vi "watt_decluster_by_time.vi"(9 "t_final":dbl format="%_19f", 10 "t_init":dbl format="%_19f", 11 "watt array cluster":T1) -> (2 "Dados":dbl[][](array[numeric]), 3 "Tempo":dbl[](array[numeric]))   [LabVIEW 2019]
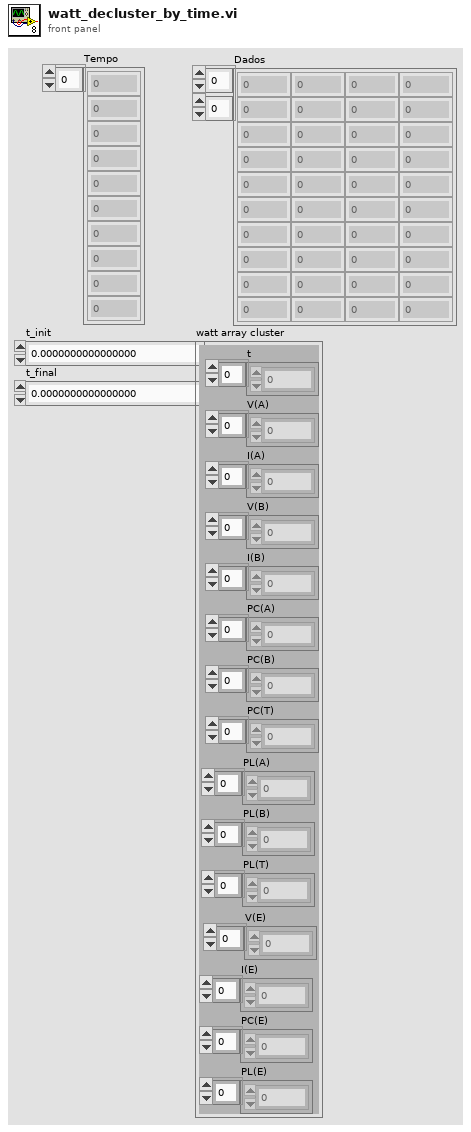
[diagram p1: front panel]
types:
  T1 = cluster{"t":dbl[], "V(A)":dbl[], "I(A)":dbl[], "V(B)":dbl[], "I(B)":dbl[], "PC(A)":dbl[], "PC(B)":dbl[], "PC(T)":dbl[], "PL(T)":dbl[], "PL(B)":dbl[], "PL(A)":dbl[], "V(E)":dbl[], "PL(E)":dbl[], "PC(E)":dbl[], "I(E)":dbl[]}
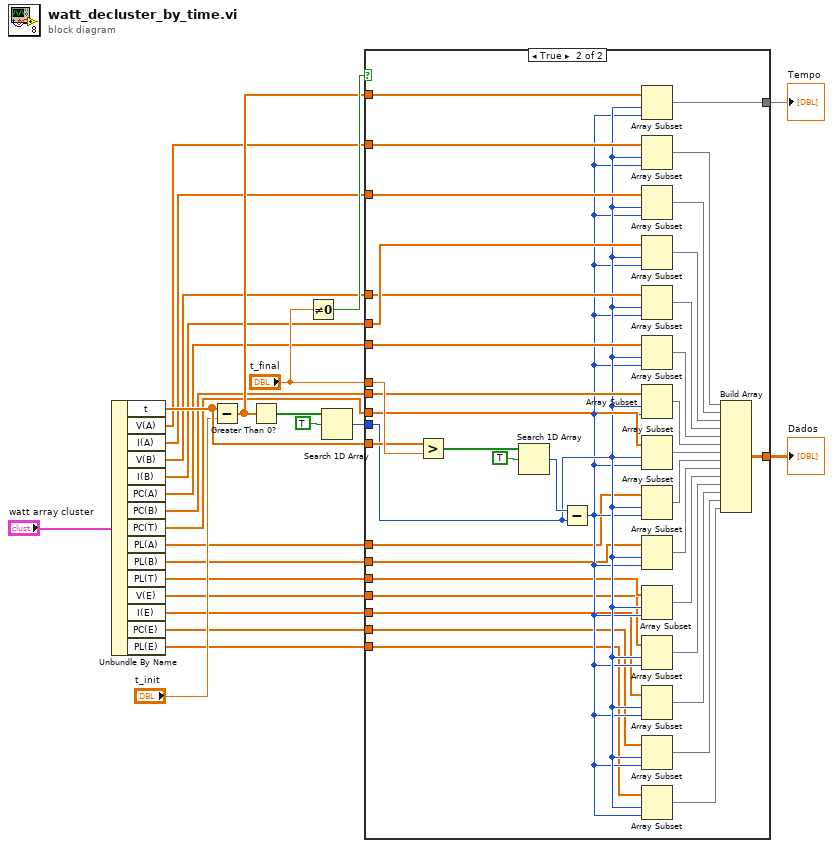
[diagram p0: block diagram]
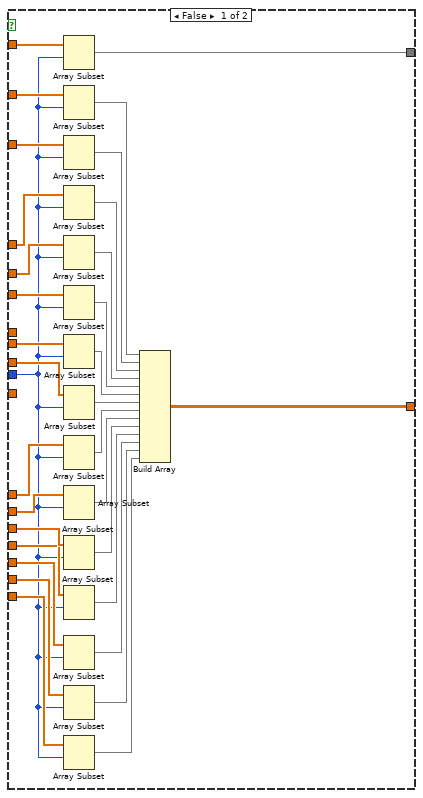
[diagram p2: hidden frame]
diagram:
  n1 = Unbundle By Name("watt array cluster") -> ("t"=w19:dbl[], "V(A)"=w13:dbl[], "I(A)"=w14:dbl[], "V(B)"=w16:dbl[], "I(B)"=w15:dbl[], "PC(A)"=w11:dbl[], "PC(B)"=w10:dbl[], "PC(T)"=w9:dbl[], "PL(A)"=w7:dbl[], "PL(B)"=w6:dbl[], "PL(T)"=w5:dbl[], "V(E)"=w4:dbl[], "I(E)"=w3:dbl[], "PC(E)"=w2:dbl[], "PL(E)"=w1:dbl[])
  n2 = Subtract(x=w19, y="t_init") -> (x-y=w22:dbl[])
  n3 = Greater Than 0?(x=w22) -> (x > 0?=w24:bool[])
  n4 = Not Equal To 0?(x="t_final") -> (x != 0?=w23:bool)
  n5 = Search 1D Array(1D array=w24, element=TRUE) -> (index of element=w21:i32)  [unwired: 1 in]
  n6 = case shown="True" w23 {
    tunnel: w22 -> [w57 w95]
    tunnel: w21 -> [w33 w73]
    tunnel: [w56 w94] -> w20
    tunnel: "t_final" -> [_ w90]
    tunnel: w19 -> [_ w89]
    tunnel: w16 -> [w51 w81]
    tunnel: w15 -> [w50 w82]
    tunnel: w14 -> [w49 w83]
    tunnel: w13 -> [w48 w84]
    tunnel: [w47 w80] -> w12
    tunnel: w11 -> [w46 w79]
    tunnel: w10 -> [w45 w78]
    tunnel: w9 -> [w44 w77]
    tunnel: w7 -> [w40 w71]
    tunnel: w6 -> [w39 w70]
    tunnel: w5 -> [w38 w69]
    tunnel: w4 -> [w37 w68]
    tunnel: w3 -> [w36 w67]
    tunnel: w2 -> [w35 w66]
    tunnel: w1 -> [w34 w65]
    frame False {
      n7 = Array Subset(array=w57, index=w33) -> (w56:dbl[])  [unwired: 1 in]
      n8 = Array Subset(array=w48, index=w33) -> (w52:dbl[])  [unwired: 1 in]
      n9 = Array Subset(array=w49, index=w33) -> (w53:dbl[])  [unwired: 1 in]
      n10 = Array Subset(array=w51, index=w33) -> (w54:dbl[])  [unwired: 1 in]
      n11 = Array Subset(array=w50, index=w33) -> (w55:dbl[])  [unwired: 1 in]
      n12 = Array Subset(array=w46, index=w33) -> (w43:dbl[])  [unwired: 1 in]
      n13 = Array Subset(array=w45, index=w33) -> (w42:dbl[])  [unwired: 1 in]
      n14 = Array Subset(array=w44, index=w33) -> (w41:dbl[])  [unwired: 1 in]
      n15 = Array Subset(array=w40, index=w33) -> (w32:dbl[])  [unwired: 1 in]
      n16 = Array Subset(array=w39, index=w33) -> (w31:dbl[])  [unwired: 1 in]
      n17 = Array Subset(array=w38, index=w33) -> (w30:dbl[])  [unwired: 1 in]
      n18 = Array Subset(array=w37, index=w33) -> (w29:dbl[])  [unwired: 1 in]
      n19 = Array Subset(array=w36, index=w33) -> (w28:dbl[])  [unwired: 1 in]
      n20 = Array Subset(array=w35, index=w33) -> (w27:dbl[])  [unwired: 1 in]
      n21 = Array Subset(array=w34, index=w33) -> (w26:dbl[])  [unwired: 1 in]
      n22 = Build Array(w52, w53, w54, w55, w43, w42, w41, w32, w31, w30, w29, w28, w27, w26) -> (w47:dbl[][])
    }
    frame True {
      n23 = Greater?(x=w89, y=w90) -> (0:w92:bool[])
      n24 = Search 1D Array(1D array=w92, element=TRUE) -> (index of element=w93:i32)  [unwired: 1 in]
      n25 = Subtract(x=w93, y=w73) -> (x-y=w72:i32)
      n26 = Array Subset(array=w95, index=w73, length=w72) -> (w94:dbl[])
      n27 = Array Subset(array=w84, index=w73, length=w72) -> (w85:dbl[])
      n28 = Array Subset(array=w83, index=w73, length=w72) -> (w86:dbl[])
      n29 = Array Subset(array=w82, index=w73, length=w72) -> (w87:dbl[])
      n30 = Array Subset(array=w81, index=w73, length=w72) -> (w88:dbl[])
      n31 = Array Subset(array=w79, index=w73, length=w72) -> (w76:dbl[])
      n32 = Array Subset(array=w78, index=w73, length=w72) -> (w75:dbl[])
      n33 = Array Subset(array=w77, index=w73, length=w72) -> (w74:dbl[])
      n34 = Array Subset(array=w71, index=w73, length=w72) -> (w64:dbl[])
      n35 = Array Subset(array=w70, index=w73, length=w72) -> (w63:dbl[])
      n36 = Array Subset(array=w69, index=w73, length=w72) -> (w62:dbl[])
      n37 = Array Subset(array=w68, index=w73, length=w72) -> (w61:dbl[])
      n38 = Array Subset(array=w67, index=w73, length=w72) -> (w60:dbl[])
      n39 = Array Subset(array=w66, index=w73, length=w72) -> (w59:dbl[])
      n40 = Array Subset(array=w65, index=w73, length=w72) -> (w58:dbl[])
      n41 = Build Array(w85, w86, w87, w88, w76, w75, w74, w64, w63, w62, w61, w60, w59, w58) -> (w80:dbl[][])
    }
  }
  "Tempo" <- w20
  "Dados" <- w12
